vi "Heater Recipe Editor.vi"() -> ()   [LabVIEW 2020]
uses:
  Recipe Entry/Data.ctl
  ControlArray/ControlArray/Step Info.ctl
  Recipe Entry/Recipe Entry.xctl
  ControlArray/ControlArray/Event Prefs.ctl
  ControlArray/ControlArray/ControlArray.lvclass
panel:
  out "Preview":cluster{"X":dbl, "Y":dbl}[](graph)
  in  "Recipe Entry 4":cluster{"Step Info":T1, "Remove":bool}(xcontrol)
  in  "Recipe Entry 3":cluster{"Step Info":T1, "Remove":bool}(xcontrol)
  in  "Recipe Entry 2":cluster{"Step Info":T1, "Remove":bool}(xcontrol)
  in  "Recipe Entry 1":cluster{"Step Info":T1, "Remove":bool}(xcontrol)
  in  "Add":bool
  in  "Array":T2[](array[typedef])
  in  "Scrollbar":i32(c297)
  # "Target\n(°F)"
  # "Duration\n(HH:MM)"
  # "This array should normally be out of view or hidden. It's visible here for demonstration but it is not intended to be interacted with outside of the library's API. It is (or should be) safe to read from the array."
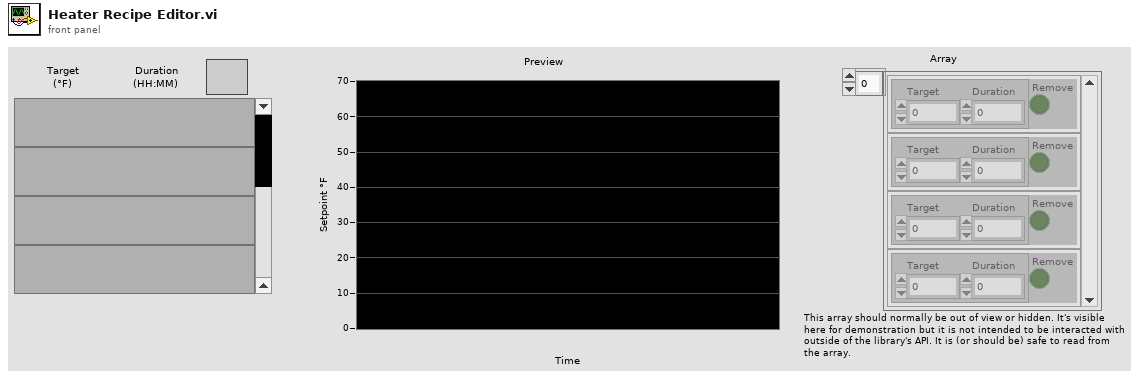
[diagram p1: front panel]
types:
  T1 = typedef "Step Info.ctl" = cluster{"Target":dbl, "Duration":dbl}
  T2 = typedef "Recipe Entry.xctl/Data.ctl" = cluster{"Step Info":T1, "Remove":bool}
  T3 = typedef "Control Array.lvlib/ControlArray.lvclass/Event Prefs.ctl" = cluster{"Mouse Wheel Scroll":bool}
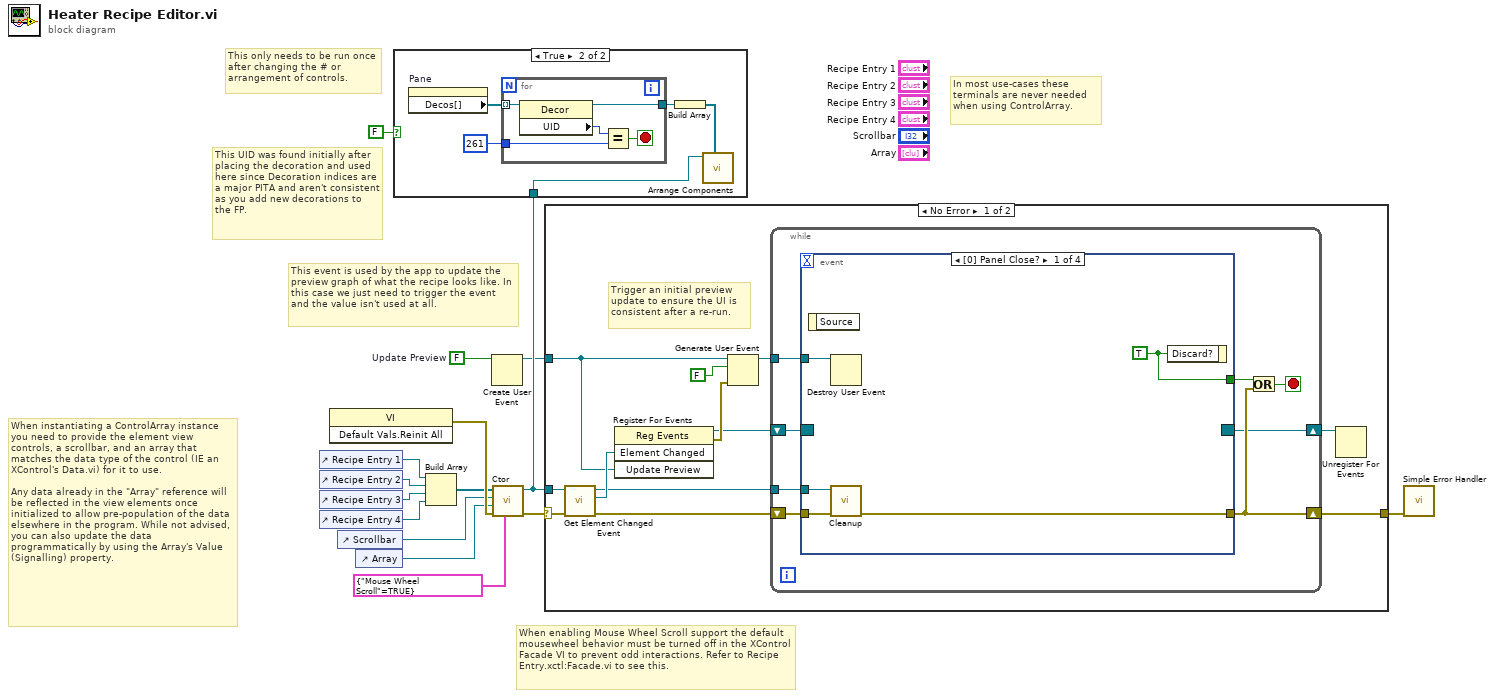
[diagram p0: block diagram]
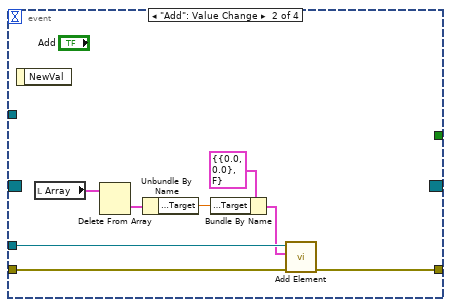
[diagram p2: hidden frame]
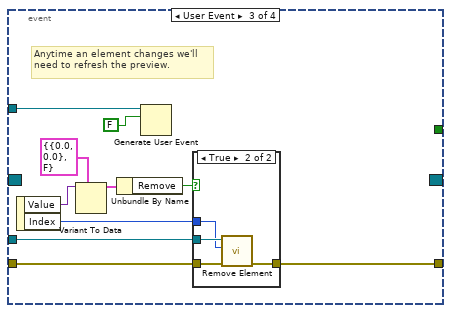
[diagram p3: hidden frame]
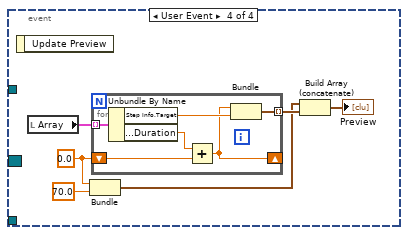
[diagram p5: hidden frame]
diagram:
  w3 = FALSE  # Update Preview
  # "This event is used by the app to update the preview graph of what the recipe looks like. In this case we just need to trigger the event and the value isn't used at all."
  # "This UID was found initially after placing the decoration and used here since Decoration indices are a major PITA and aren't consistent as you add new decorations to the FP."
  # "In most use-cases these terminals are never needed when using ControlArray."
  # "When instantiating a ControlArray instance you need to provide the element view controls, a scrollbar, and an array that matches the data type of the control (IE an XControl's Data.vi) for it to use.\n\nAny data already in the \"Array\" reference will be reflected in the view elements once initialized to allow pre-population of the data elsewhere in the program. While not advised, you can also update the data programmatically by using the Array's Value (Signalling) property."
  # "When enabling Mouse Wheel Scroll support the default mousewheel behavior must be turned off in the XControl Facade VI to prevent odd interactions. Refer to Recipe Entry.xctl:Facade.vi to see this."
  # "This only needs to be run once after changing the # or arrangement of controls."
  n1 = control-ref of="Recipe Entry 1"() -> (w8:refnum<vi>)
  n2 = control-ref of="Recipe Entry 2"() -> (w9:refnum<vi>)
  n3 = control-ref of="Recipe Entry 3"() -> (w10:refnum<vi>)
  n4 = control-ref of="Recipe Entry 4"() -> (w7:refnum<vi>)
  n5 = invoke class="VI" method="Default Vals.Reinit All"() -> (error out=w15:errorcluster)  [unwired: 3 in, 2 out]
  n6 = control-ref of="Scrollbar"() -> (w13:refnum<vi>)
  n7 = control-ref of="Array"() -> (w12:refnum<vi>)
  n8 = Build Array(w8, w9, w10, w7) -> (w14:refnum<vi>[])
  n9 = Create User Event(user event datatype=w3) -> (user event=w2:refnum<user-event>)  [unwired: 1 in, 1 out]
  n10 = call "Ctor.vi"("Event Prefs"=T3 {"Mouse Wheel Scroll"=TRUE}, "error in (no error)"=w15, "Array"=w12, "Scrollbar"=w13, "Controls"=w14) -> ("error out"=w4:errorcluster, "ControlArray out"=w5:refnum<class "ControlArray.lvclass">)  [unwired: 5 in]
  n11 = case shown="True" FALSE {
    tunnel: w5 -> [_ w20]
    frame False {
    }
    frame True {
      n12 = property on="Pane" class="Pane"() -> ("Decos[]"=w18:refnum<vi>[])  [unwired: 2 in, 2 out]
      n13 = for {
        tunnel: w18 -> [w25] mode=indexing
        tunnel: [w24] -> w17
        tunnel: 261 ("UID") -> [w21]
        stop <- w23 stop-if-true
        n14 = property class="Decor"(reference=w25) -> (reference out=w24:refnum<vi>, "UID"=w22:i32)  [unwired: 1 in, 1 out]
        n15 = Equal?(x=w22, y=w21) -> (x = y?=w23:bool)
      }
      n16 = Build Array(w17) -> (w19:refnum<vi>[])
      n17 = call "Arrange Components.vi"("Decos"=w19, "ControlArray"=w20) -> ()  [unwired: 9 in, 1 out]
    }
  }
  n18 = case shown="No Error" w4 {
    selector: w4 -> [w35 w85]
    tunnel: [w34 w85] -> w6
    tunnel: w5 -> [w32 _]
    tunnel: w2 -> [w28 _]
    frame No Error {
      # "Trigger an initial preview update to ensure the UI is consistent after a re-run."
      n19 = call "Get Element Changed Event.vi"("ControlArray in"=w32) -> ("Element Changed"=w33:refnum<user-event>, "ControlArray out"=w30:refnum<class "ControlArray.lvclass">)  [unwired: 8 in, 1 out]
      n20 = register-events(w33, w28) -> (reference out=w31:refnum<event-registration>, error out=w36:errorcluster)  [unwired: 2 in]
      n21 = Generate User Event(user event=w28, event data cluster=FALSE, error in=w36) -> (user event out=w27:refnum<user-event>)  [unwired: 1 in, 1 out]
      n22 = while {
        shift-right: [w42] -> w29
        shift-left: w31 -> [w43]
        tunnel: w30 -> [w40]
        shift-right: [w44] -> w34
        shift-left: w35 -> [w39]
        tunnel: w27 -> [w37]
        stop <- w38 stop-if-true
        n23 = event shown="[0] Panel Close?" {
          selector: w43 -> [_ _ _ _]
          dyn-events: [_ _ _ _] -> w42
          timeout: _ -> [_ _ _ _]
          tunnel: [w49 _ _ _] -> w41
          tunnel: w40 -> [w48 w57 w62 _]
          tunnel: w39 -> [w47 w56 w61 _]
          tunnel: [w46 w55 w58 _] -> w44
          tunnel: w37 -> [w45 _ w60 _]
          event Panel Close? {
            w49 = TRUE ("Discard?")
            n24 = event-data() -> ()  [unwired: 1 in, 1 out]
            n25 = Destroy User Event(user event=w45) -> ()  [unwired: 1 in, 1 out]
            n26 = call "Cleanup.vi"("error in (no error)"=w47, "ControlArray in"=w48) -> ("error out"=w46:errorcluster)  [unwired: 9 in]
            n27 = event-data("Discard?"=w49) -> ()  [unwired: 1 in, 1 out]
          }
          event "Add": Value Change {
            n28 = event-data() -> ()  [unwired: 1 in, 1 out]
            n29 = local read "Array"() -> (w53:T2[])
            n30 = Delete From Array(array=w53) -> (deleted portion=w52:T2)  [unwired: 2 in, 1 out]
            n31 = Unbundle By Name(w52) -> ("Step Info.Target"=w51:dbl)
            n32 = Bundle By Name(cluster=T2 {"Step Info"={"Target"=0.0, "Duration"=0.0}, "Remove"=FALSE} ("Recipe Entry"), "Step Info.Target"=w51) -> (w50:T2)
            n33 = call "Add Element.vi"("error in (no error)"=w56, "Value"=w50, "ControlArray in"=w57) -> ("error out"=w55:errorcluster)  [unwired: 7 in, 1 out]
          }
          event User Event {
            # "Anytime an element changes we'll need to refresh the preview."
            n34 = event-data() -> ("Value"=w67:variant, "Index"=w64:i32)  [unwired: 1 in]
            n35 = Variant To Data(type=T2 {"Step Info"={"Target"=0.0, "Duration"=0.0}, "Remove"=FALSE} ("Recipe Entry"), Variant=w67) -> (data=w63:T2)  [unwired: 1 in, 1 out]
            n36 = Unbundle By Name(w63) -> ("Remove"=w65:bool)
            n37 = Generate User Event(user event=w60, event data cluster=FALSE) -> ()  [unwired: 2 in, 2 out]
            n38 = case shown="True" w65 {
              tunnel: w64 -> [_ w70]
              tunnel: w62 -> [_ w72]
              tunnel: w61 -> [w68 w71]
              tunnel: [w68 w69] -> w58
              frame False {
              }
              frame True {
                n39 = call "Remove Element.vi"("error in (no error)"=w71, "Index"=w70, "ControlArray in"=w72) -> ("error out"=w69:errorcluster)  [unwired: 6 in, 2 out]
              }
            }
          }
          event User Event {
            w76 = 0.0
            n40 = event-data() -> ()  [unwired: 1 in, 1 out]
            n41 = local read "Array"() -> (w78:T2[])
            n42 = Bundle(w76, 70.0) -> (w74:cluster{dbl, dbl})  [unwired: 1 in]
            n43 = for {
              tunnel: w78 -> [w84] mode=indexing
              shift-right: [w80] -> _
              shift-left: w76 -> [w82]
              tunnel: [w79] -> w75 mode=indexing
              n44 = Unbundle By Name(w84) -> ("Step Info.Target"=w83:dbl, "Step Info.Duration"=w81:dbl)
              n45 = Add(x=w81, y=w82) -> (x+y=w80:dbl)
              n46 = Bundle(w80, "Target"=w83) -> (w79:cluster{dbl, "Target":dbl})  [unwired: 1 in]
            }
            n47 = Build Array (concatenate)(w74, w75) -> (→"Preview":cluster{dbl, "Target":dbl}[])
          }
        }
        n48 = Or(x=w41, y=w44) -> (x .or. y?=w38:bool)
      }
      n49 = Unregister For Events(event registration refnum=w29) -> ()  [unwired: 1 in, 1 out]
    }
    frame Error {
    }
  }
  n50 = call <vilib>:"Simple Error Handler.vi"("error in (no error)"=w6) -> ()  [unwired: 4 in, 5 out]
